vi "ITR HP order 2.vi"(7 "input":dbl format="%.2f", 13 "corner period (steps)":dbl(slide)=10.237739663395852 scale=1.0..1000.0) -> (8 "output":dbl format="%.2f")   [LabVIEW 2016]
doc: "Modular ITR second order high pass filter with internal shift registers.\n\nAlexis Lopez\nP350\nCSUSB Physics"
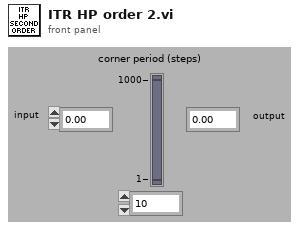
[diagram p1: front panel]
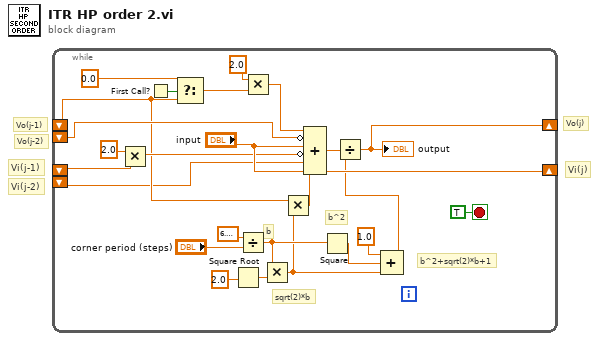
[diagram p0: block diagram]
diagram:
  # "Vo(j-2)"
  # "Vi(j-2)"
  # "Vi(j-1)"
  # "Vi(j)"
  # "Vo(j-1)"
  # "Vo(j)"
  n1 = while {
    shift-left: _ -> [w4]
    shift-right: [w22] -> _
    shift-right: ["input"] -> _
    shift-left: _ -> [w17]
    shift-left: _ -> [w11]
    shift-left: _ -> [w2]
    stop <- TRUE stop-if-true
    # "b^2"
    # "sqrt(2)*b"
    # "b^2+sqrt(2)*b+1"
    # "b"
    n2 = Multiply(x=2.0, y=w17) -> (x*y=w15:dbl)
    n3 = First Call?() -> (First Call?: T/F=w21:bool)
    n4 = Select(t=0.0, s=w21, f=w4) -> (s? t:f=w14:dbl)
    n5 = Square Root(x=2.0) -> (sqrt(x)=w8:dbl)
    n6 = Divide(x=6.283185307179586, y="corner period (steps)") -> (x/y=w9:dbl)
    n7 = Multiply(x=2.0, y=w14) -> (x*y=w12:dbl)
    n8 = Multiply(x=w9, y=w8) -> (x*y=w3:dbl)
    n9 = Multiply(x=w4, y=w3) -> (x*y=w1:dbl)
    n10 = Compound Arithmetic op=ADD(w12, invert w11, "input", invert w15, w2, w1) -> (w18:dbl)
    n11 = Square(x=w9) -> (x^2=w7:dbl)
    n12 = Compound Arithmetic op=ADD(1.0 ("t"), w7, w3) -> (w5:dbl)
    n13 = Divide(x=w18, y=w5) -> (x/y=w22:dbl)
    "output" <- w22
  }
